vi "InitLeonardoAsJoystick.vi"() -> (0 "error out":errorcluster, 3 "Refnum out":refnum<k1>)   [LabVIEW 2014]
doc: "find the Arduino Leonardo among all plugged in joystick and initialize it"
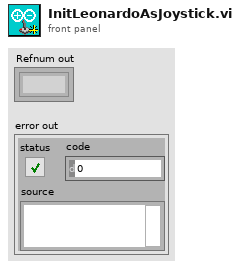
[diagram p1: front panel]
types:
  T1 = cluster{"axes total":u32, "buttons total":u32, "pov total":u32, "device name":string}[]
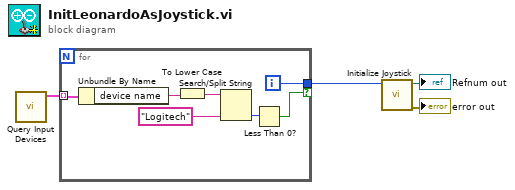
[diagram p0: block diagram]
diagram:
  n1 = call <vilib>:"Query Input Devices.vi"() -> ("joystick info"=w3:T1)  [unwired: 8 in, 3 out]
  n2 = for {
    tunnel: w3 -> [w11] mode=indexing
    tunnel: [w7] -> w4 if=w5
    i -> [w7]
    n3 = Unbundle By Name(w11) -> ("device name"=w10:string)
    n4 = To Lower Case(string=w10) -> (all lower case string=w9:string)
    n5 = Search/Split String(string=w9, search string/char (-)="Logitech") -> (offset of match=w6:i32)  [unwired: 1 in, 2 out]
    n6 = Less Than 0?(x=w6) -> (x < 0?=w5:bool)
  }
  n7 = call <vilib>:"Initialize Joystick.vi"("device index"=w4) -> ("error out"=→"error out":errorcluster, "device ID"=→"Refnum out":refnum<k1>)  [unwired: 9 in]
